vi "sendScript.vi"(8 "error in (no error)":errorcluster, 11 "K2602 in":refnum<class "K2602.lvclass">) -> (0 "error out":errorcluster, 3 "K2602 out":refnum<class "K2602.lvclass">)   [LabVIEW 2009, in "Hardware.lvlib" / "Channels.lvlib" / "K2602.lvclass"]
uses:
  K2602.lvclass
  K2602.lvclass/K2602.ctl
  <instrlib>/Keithley 2600 Series/Keithley 2600 Series.lvlib
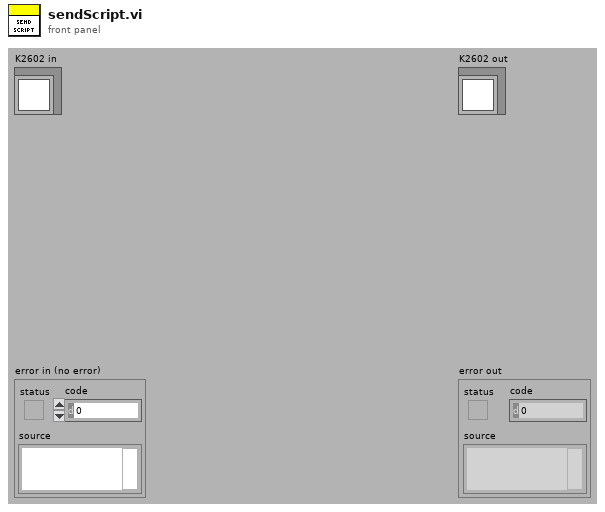
[diagram p1: front panel]
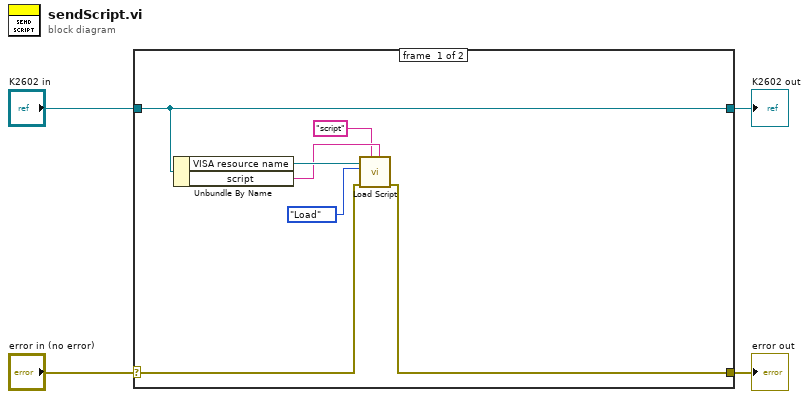
[diagram p0: block diagram]
diagram:
  n1 = case shown="No Error" "error in (no error)" {
    selector: "error in (no error)" -> [w8 w13]
    tunnel: [w7 w13] -> w3
    tunnel: [w11 w12] -> w1
    tunnel: "K2602 in" -> [w11 w12]
    frame #0 {
      n2 = Unbundle By Name(w11) -> ("VISA resource name"=w10:refnum<visa-resource-name>, "script"=w6:string)
      n3 = call <instrlib>:"Load Script.vi"("Script"=w6, "Script Name"="script", "error in"=w8, "Load Options (Load)"=enum16{"Load", "Load & Run"}."Load", "VISA resource name"=w10) -> ("error out"=w7:errorcluster)  [unwired: 4 in, 2 out]
    }
    frame #1 {
    }
  }
  "error out" <- w3
  "K2602 out" <- w1
